vi "Get Range.vi"(8 "error in (no error)":errorcluster, 11 "MCListbox with Checkboxes in":refnum<class "MCListbox with Checkboxes.lvclass">) -> (0 "error out":errorcluster, 2 "Range":cluster{"Rows":i32, "Columns":i32}, 3 "MCListbox with Checkboxes out":refnum<class "MCListbox with Checkboxes.lvclass">)   [LabVIEW 2016, in "MCListbox with Checkboxes.lvclass"]
uses:
  MCListbox with Checkboxes.lvclass
  MCListbox with Checkboxes.lvclass/MCListbox with Checkboxes.ctl
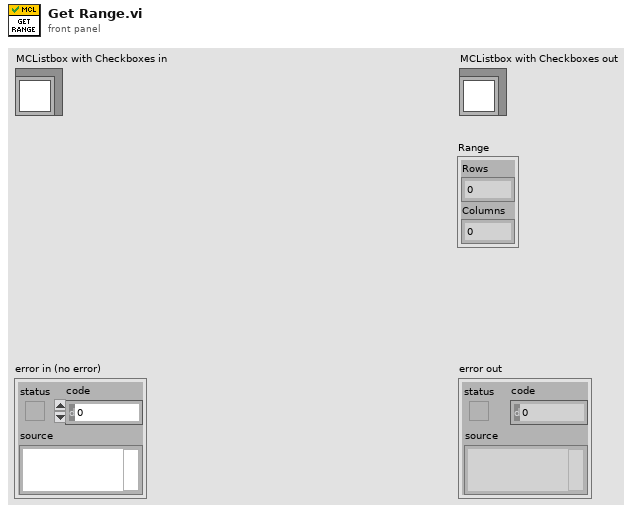
[diagram p1: front panel]
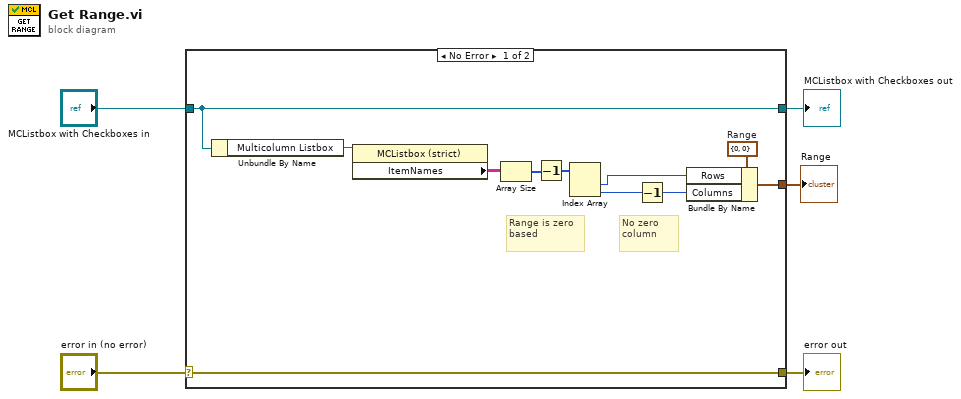
[diagram p0: block diagram]
diagram:
  n1 = case shown="No Error" "error in (no error)" {
    selector: "error in (no error)" -> [w16 w18]
    tunnel: [w16 w18] -> w4
    tunnel: [w15 w17] -> w2
    tunnel: "MCListbox with Checkboxes in" -> [w15 w17]
    tunnel: [w8 _] -> w1
    frame No Error {
      w12 = cluster{"Rows":i32, "Columns":i32} {"Rows"=0, "Columns"=0}  # Range
      # "Range is zero based"
      # "No zero column"
      n2 = Unbundle By Name(w15) -> ("Multicolumn Listbox"=w14:refnum<vi>)
      n3 = property class="MCListbox (strict)"(reference=w14) -> ("ItemNames"=w13:string[][])  [unwired: 1 in, 2 out]
      n4 = Array Size(array=w13) -> (size(s)=w11:i32[])
      n5 = Decrement(x=w11) -> (x-1=w6:i32[])
      n6 = Index Array(array=w6) -> (element #1=w10:i32, element #2=w9:i32)  [unwired: 2 in]
      n7 = Decrement(x=w9) -> (x-1=w7:i32)
      n8 = Bundle By Name(cluster=w12, "Rows"=w10, "Columns"=w7) -> (w8:cluster{"Rows":i32, "Columns":i32})
    }
    frame Error {
    }
  }
  "error out" <- w4
  "MCListbox with Checkboxes out" <- w2
  "Range" <- w1
